vi "Send String to Com Port.vi"(8 "error in (no error)":errorcluster, 9 "Wait after Msecs":dbl, 10 "String":string, 11 "VISA resource name":refnum<visa-resource-name>) -> (0 "error out":errorcluster, 3 "VISA resource name 2":refnum<visa-resource-name>)   [LabVIEW 2013]
panel:
  # "This progarm seperates out strings of commands into single\ncharacters and writes them to the buffer one at a time.  Last I\nchecked, this worked fine.  It is possible that this may not be \nneeded in the future."
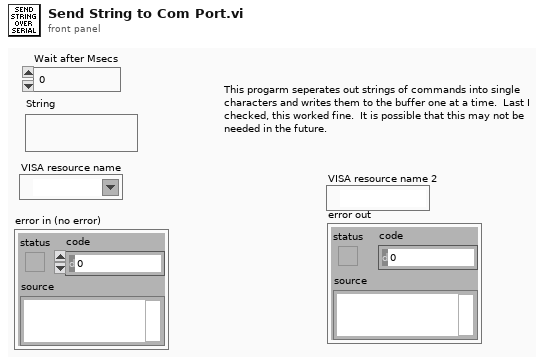
[diagram p1: front panel]
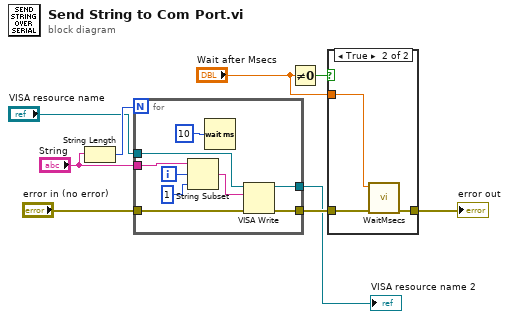
[diagram p0: block diagram]
diagram:
  n1 = String Length(string="String") -> (length=w9:i32)
  n2 = for {
    N: w9 -> [_]
    tunnel: "String" -> [w18]
    tunnel: "VISA resource name" -> [w15]
    tunnel: "error in (no error)" -> [w14]
    tunnel: [w13] -> w1
    tunnel: [w12] -> w3
    i -> [w17]
    n3 = String Subset(string=w18, offset (0)=w17, length (rest)=1 ("length (rest)")) -> (substring=w11:string)
    n4 = Wait (ms)(milliseconds to wait=u32 10) -> ()  [unwired: 1 out]
    n5 = VISA Write(VISA resource name=w15, write buffer=w11, error in (no error)=w14) -> (VISA resource name out=w13:refnum<visa-resource-name>, error out=w12:errorcluster)  [unwired: 1 out]
  }
  "VISA resource name 2" <- w1
  n6 = Not Equal To 0?(x="Wait after Msecs") -> (x != 0?=w5:bool)
  n7 = case shown="True" w5 {
    tunnel: "Wait after Msecs" -> [_ w22]
    tunnel: w3 -> [w19 w21]
    tunnel: [w19 w20] -> w2
    frame False {
    }
    frame True {
      n8 = call "WaitMsecs.vi"("error in (no error)"=w21, "Wait Msecs"=w22) -> ("error out"=w20:errorcluster)  [unwired: 9 in]
    }
  }
  "error out" <- w2
